vi "ButtonMotorControl.vi"(6 "Allow Down":bool, 7 "Allow Up":bool, 9 "Down":bool, 10 "Up":bool, 11 "Speed":dbl) -> (3 "Motor Speed":dbl)   [LabVIEW 2014]
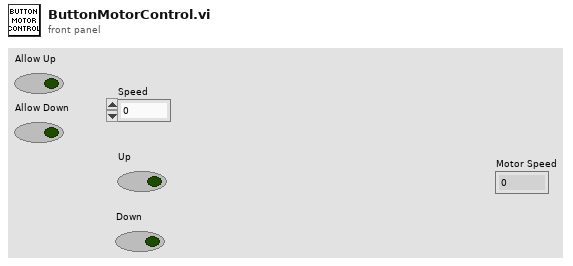
[diagram p1: front panel]
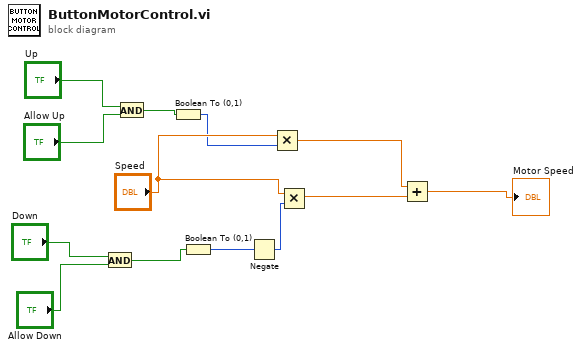
[diagram p0: block diagram]
diagram:
  n1 = And(x="Down", y="Allow Down") -> (x .and. y?=w1:bool)
  n2 = And(x="Up", y="Allow Up") -> (x .and. y?=w4:bool)
  n3 = Boolean To (0,1)(Boolean=w4) -> (0, 1=w9:i16)
  n4 = Boolean To (0,1)(Boolean=w1) -> (0, 1=w8:i16)
  n5 = Negate(x=w8) -> (-x=w7:i16)
  n6 = Multiply(x="Speed", y=w9) -> (x*y=w12:dbl)
  n7 = Multiply(x="Speed", y=w7) -> (x*y=w11:dbl)
  n8 = Add(x=w12, y=w11) -> (x+y=→"Motor Speed":dbl)
